vi "FPGA_GlobalOpen.vi"(8 "error in (no error)":errorcluster) -> (0 "error out":errorcluster, 3 "GlobalDevRef":T1)   [LabVIEW 2017]
uses:
  <vilib>/Rock Robotics/SystemInterfaces/Global/FPGA_GlobalDevRef.ctl
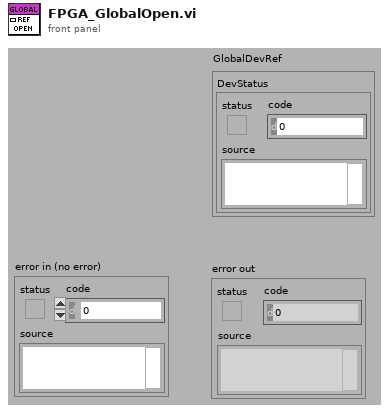
[diagram p1: front panel]
types:
  T1 = typedef "FPGA_GlobalDevRef.ctl" = cluster{"DevStatus":errorcluster}
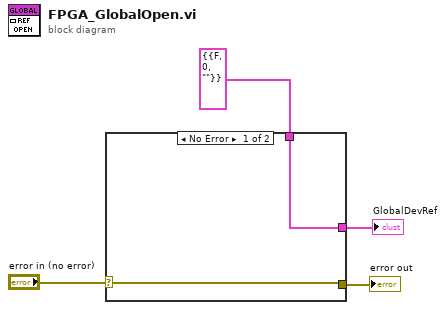
[diagram p0: block diagram]
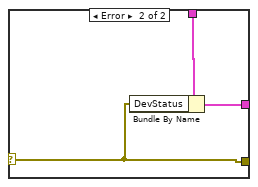
[diagram p2: hidden frame]
diagram:
  n1 = case shown="No Error" "error in (no error)" {
    selector: "error in (no error)" -> [w5 w7]
    tunnel: T1 {"DevStatus"={"status"=FALSE, "code"=0, "source"=""}} ("GlobalDevRef") -> [w6 w9]
    tunnel: [w6 w8] -> w3
    tunnel: [w5 w7] -> w1
    frame No Error {
    }
    frame Error {
      n2 = Bundle By Name(cluster=w9, "DevStatus"=w7) -> (w8:T1)
    }
  }
  "GlobalDevRef" <- w3
  "error out" <- w1
